vi "itemIcon.vi"(8 "Error In":errorcluster, 10 "index":i32, 11 "QToolBox In":refnum<class "QToolBox.lvclass">) -> (0 "Error Out":errorcluster, 2 "Value":refnum<class "QIcon.lvclass">, 3 "QToolBox Out":refnum<class "QToolBox.lvclass">)   [LabVIEW 2014, in "QToolBox.lvclass"]
doc: "LabVIEW-specific documentation is not yet available. See <b>https://doc.qt.io/qt-5/qtoolbox.html#itemIcon</b>"
uses:
  QToolBox.lvclass
  Qt GUI/QIcon/QIcon.lvclass
  LQ Core/LQIdentity/LQIdentity.lvclass/LQIdentity.ctl
  LQ Core/LQSerialData/LQSerialData.lvclass/LQSerialData.ctl
  LQ Core/LQ Core.lvlib
  LQ Core/LQIdentity/LQIdentity.lvclass
  LQ Core/LQSerialData/LQSerialData.lvclass
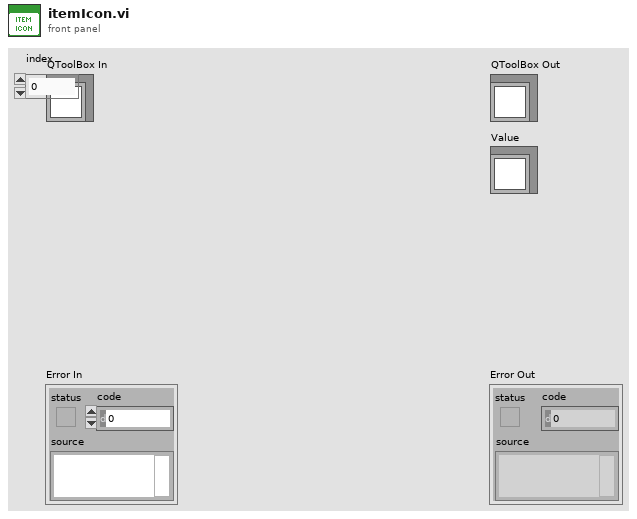
[diagram p1: front panel]
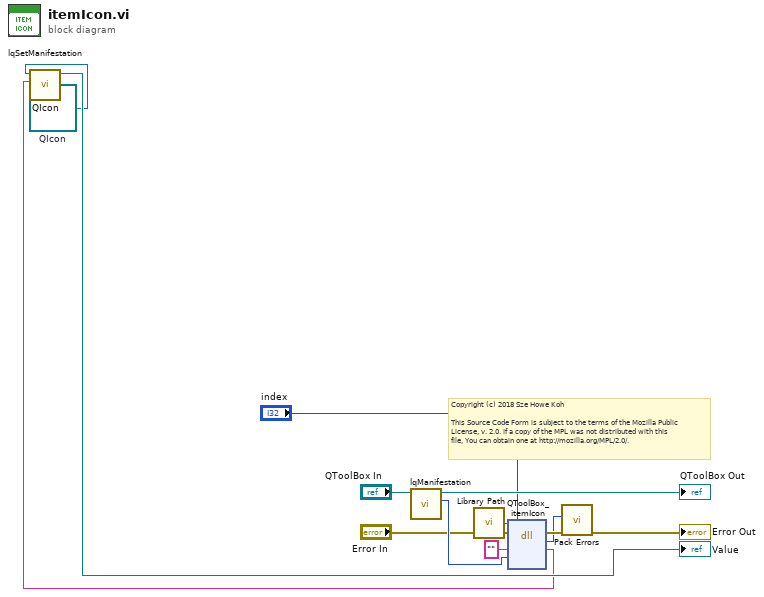
[diagram p0: block diagram]
diagram:
  w2 = refnum<class "QIcon.lvclass"> refnum  # QIcon
  # "Copyright (c) 2018 Sze Howe Koh\n\nThis Source Code Form is subject to the terms of the Mozilla Public\nLicense, v. 2.0. If a copy of the MPL was not distributed with this\nfile, You can obtain one at http://mozilla.org/MPL/2.0/."
  n1 = call "lqManifestation.vi"("LQIdentity in"="QToolBox In") -> ("Manifestation"=w9:u64, "LQIdentity out"=→"QToolBox Out":refnum<class "QToolBox.lvclass">)  [unwired: 9 in]
  n2 = call "Library Path.vi"() -> ("Library Path"=w10:path)
  n3 = dll-call lib="?" fn="QToolBox_itemIcon"(path in=w10, error in="Error In", "_retVal"="" ("retVal"), "_instance"=w9, "index"="index") -> (error out=w7:errorcluster, w5:i32, "_retVal"=w3:string)  [unwired: 3 in, 1 out]
  n4 = call "lqSetManifestation.vi"("Manifestation"=w3, "LQSerialData in"=w2) -> ("LQSerialData out"=→"Value":refnum<class "QIcon.lvclass">)  [unwired: 8 in, 1 out]
  n5 = call "Pack Errors.vi"("Error In"=w7, "Error Code"=w5) -> ("Error Out"=→"Error Out":errorcluster)  [unwired: 9 in]
